vi "getLineStyle.vi"(0 "reference":refnum<class "SegmentedLineEdge.lvclass">, 5 "error in (no error)":errorcluster) -> (14 "reference out":refnum<class "SegmentedLineEdge.lvclass">, 15 "lineStyle":refnum<class "LineStyle.lvclass">, 19 "error out":errorcluster)   [LabVIEW 2012, in "SegmentedLineEdge.lvclass"]
doc: "public LineStyle getLineStyle()"
uses:
  <resource>/Framework/Providers/Open_GDS/UML/SegmentedLineEdge_class/SegmentedLineEdge.lvclass
  <resource>/Framework/Providers/Open_GDS/UML/LineStyle_class/LineStyle.lvclass
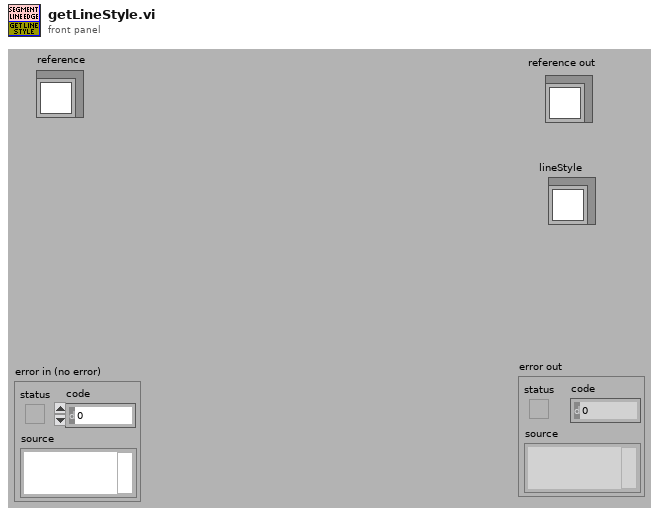
[diagram p1: front panel]
types:
  T1 = typedef "SegmentedLineEdge.lvclass/ObjectAttributes.ctl" = cluster{"lineStyle":refnum<class "LineStyle.lvclass">, "startArrowHead":refnum<class "ArrowHead.lvclass">, "endArrowHead":refnum<class "ArrowHead.lvclass">, "startLabel":string, "midLabel":string, "endLabel":string, "MidLabelOffset":T2, "SplitWire":bool}
  T2 = typedef "Point Point2D.ctl" = cluster{"x":dbl, "y":dbl}
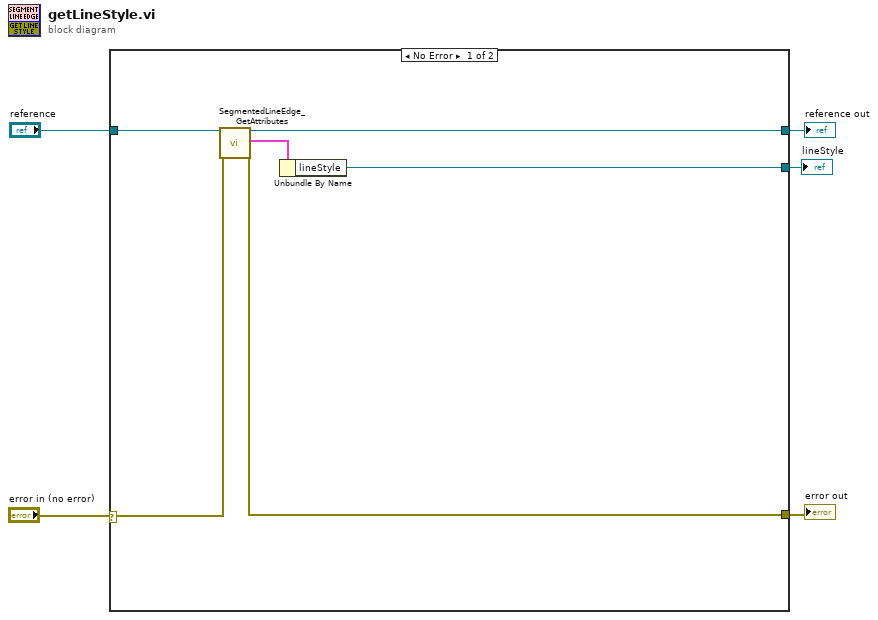
[diagram p0: block diagram]
diagram:
  n1 = case shown="No Error" "error in (no error)" {
    selector: "error in (no error)" -> [w7 w12]
    tunnel: "reference" -> [w11 w13]
    tunnel: [w10 w12] -> w4
    tunnel: [w9 w13] -> w3
    tunnel: [w8 _] -> w1
    frame No Error {
      n2 = call <resource>:"SegmentedLineEdge_GetAttributes.vi"("reference in"=w11, "error in (no error)"=w7) -> ("reference out"=w9:refnum<class "SegmentedLineEdge.lvclass">, "Data"=w6:T1, "error out"=w10:errorcluster)  [unwired: 1 in, 14 out]
      n3 = Unbundle By Name(w6) -> ("lineStyle"=w8:refnum<class "LineStyle.lvclass">)
    }
    frame Error {
    }
  }
  "reference out" <- w3
  "error out" <- w4
  "lineStyle" <- w1
